vi "Find Distances to SCM Microphones.vi"(5 "Source Polar\nCoordinates":cluster{"r":dbl, "theta":dbl}, 9 "Microphone Coordinates (cm, rad)":cluster{"r":dbl, "theta":dbl}[](array[cluster])) -> (8 "Distances (cm)":dbl[](array[numeric]))   [LabVIEW 2013]
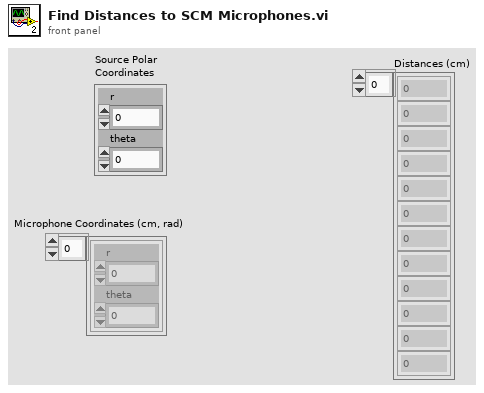
[diagram p1: front panel]
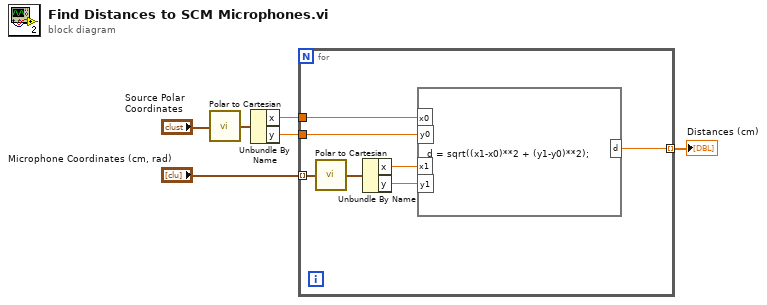
[diagram p0: block diagram]
diagram:
  n1 = call "Polar to Cartesian.vi"("Polar\nCoordinates"="Source Polar\nCoordinates") -> ("Cartesian\nCoordinates"=w4:cluster{"x":dbl, "y":dbl})  [unwired: 4 in]
  n2 = Unbundle By Name(w4) -> ("x"=w3:dbl, "y"=w2:dbl)
  n3 = for {
    tunnel: "Microphone Coordinates (cm, rad)" -> [w13] mode=indexing
    tunnel: w3 -> [w12]
    tunnel: w2 -> [w11]
    tunnel: [w7] -> w1 mode=indexing
    n4 = call "Polar to Cartesian.vi"("Polar\nCoordinates"=w13) -> ("Cartesian\nCoordinates"=w10:cluster{"x":dbl, "y":dbl})  [unwired: 4 in]
    n5 = Unbundle By Name(w10) -> ("x"=w9:dbl, "y"=w8:dbl)
    n6 = formula code="d = sqrt((x1-x0)**2 + (y1-y0)**2);"("x0"=w12, "y0"=w11, "x1"=w9, "y1"=w8) -> ("d"=w7:dbl)
  }
  "Distances (cm)" <- w1
